vi "DrawLine3D.vi"(9 "Display":T1={"Mode"=enum."Inherit Value", "PointSize"=1.0, "LineWidth"=1.0}, 10 "Color":T2={"Alpha"=1.0, "Color"=16448250} {"Alpha" min=0.0 max=1.0 scale=0.0..1.0}, 11 "Lines":cluster{"P0":T3, "P1":T3}[](array[cluster])) -> ()   [LabVIEW 2014]
uses:
  TypeDefs/Point3D.ctl
  TypeDefs/Color.ctl
  <vilib>/picture/3D Picture Control/Object/Create Object (name).vi
  <vilib>/picture/3D Picture Control/Object/Add Object (no reference).vi
  <vilib>/picture/3D Picture Control/NI_3D Picture Control.lvlib
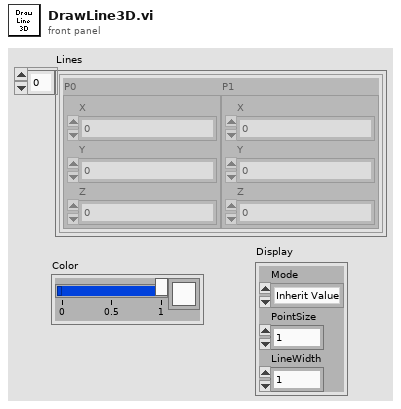
[diagram p1: front panel]
types:
  T1 = cluster{"Mode":enum16{"Inherit Value", "Points", "Wireframe", "Polygons"}, "PointSize":sgl, "LineWidth":sgl}
  T2 = typedef "Color.ctl" = cluster{"Alpha":dbl, "Color":u32}
  T3 = typedef "Point3D.ctl" = cluster{"X":sgl, "Y":sgl, "Z":sgl}
  T4 = enum16{"Points", "Lines", "Line Strip", "Line Loop", "Triangles", "Triangle Strip", "Triangle Fan", "Quads", "Quad Strip", "Polygon"}
  T5 = enum16{"New", "Find", "FindPattern", "GetTable", "Clear"}
  T6 = enum16{"Inherit Value", "Points", "Wireframe", "Polygons"}
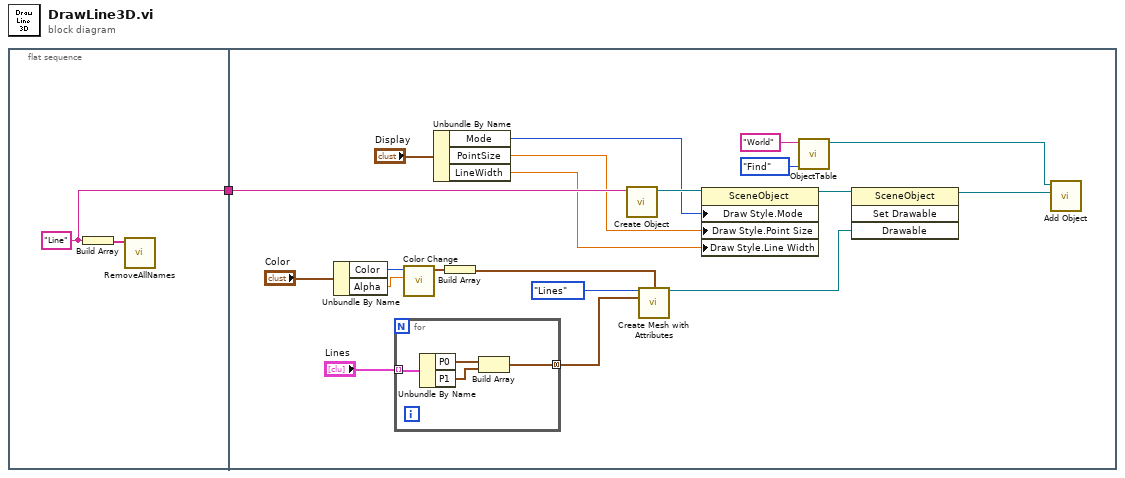
[diagram p0: block diagram]
diagram:
  n1 = flat-sequence {
    tunnel: [w2] -> w1
    tunnel: w1 -> [w8]
    frame #0 {
      w2 = "Line" ("string")
      n2 = Build Array(w2) -> (w3:string[])
      n3 = call "RemoveAllNames.vi"("Names"=w3) -> ()  [unwired: 11 in]
    }
    frame #1 {
      n4 = Unbundle By Name("Color") -> ("Color"=w14:u32, "Alpha"=w13:dbl)
      n5 = for {
        tunnel: "Lines" -> [w27] mode=indexing
        tunnel: [w24] -> w16 mode=concatenating
        n6 = Unbundle By Name(w27) -> ("P0"=w26:T3, "P1"=w25:T3)
        n7 = Build Array(w26, w25) -> (w24:T3[])
      }
      n8 = call <vilib>:"Color Change.vi"("Alpha"=w13, "Color"=w14) -> ("RGBA"=w15:cluster{"R":sgl, "G":sgl, "B":sgl, "A":sgl})  [unwired: 9 in]
      n9 = Unbundle By Name("Display") -> ("Mode"=w6:T6, "PointSize"=w5:sgl, "LineWidth"=w4:sgl)
      n10 = Build Array(w15) -> (w11:cluster{"R":sgl, "G":sgl, "B":sgl, "A":sgl}[])
      n11 = call-poly <vilib>:"Create Object.vi"("Name"=w8) -> ("Scene:New Object"=w10:refnum<vi>)  [unwired: 9 in, 1 out]
      n12 = call <vilib>:"Create Mesh with Attributes.vi"("Draw Mode"=T4."Lines", "Color Array"=w11, "Vertex Array"=w16) -> ("New Mesh Refnum"=w18:refnum<vi>)  [unwired: 11 in, 1 out]
      n13 = property class="SceneObject"(reference=w10, "Draw Style.Mode"=w6, "Draw Style.Point Size"=w5, "Draw Style.Line Width"=w4) -> (reference out=w9:refnum<vi>)  [unwired: 1 in, 1 out]
      n14 = call "ObjectTable.vi"("ObjectStoreSelector"=T5."Find", "Name"="World") -> ("ObjectRef"=w19:refnum<vi>)  [unwired: 5 in, 4 out]
      n15 = invoke class="SceneObject" method="Set Drawable"(reference=w9, "Drawable"=w18) -> (reference out=w21:refnum<vi>)  [unwired: 2 in, 3 out]
      n16 = call-poly <vilib>:"Add Object.vi"("New Object In"=w21, "Scene Object In"=w19) -> ()  [unwired: 8 in, 2 out]
    }
  }
